vi "TPNT_UpdateDevice.vi"(5 "UTC":bool, 6 "mailserver":string="localhost", 7 "tpnt_logfile":path, 8 "error in (no error)":errorcluster, 10 "Device In":T1={"device"="", "devupdate"=0.0, "next_update"=0, "devinterface"="", "TPs"=[], "Alarms"=TRUE, "monitor"=TRUE, "log sep"=""} {"TPs"."Log"."updaterate" format="%.2f"; "TPs"."Samples"."Values" format="%.2f"; "TPs"."Samples"."samples" min=1 step=1; "TPs"."Limits"."Nominal" format="%.2f"; "TPs"."Limits"."Upper" format="%.2f"; "TPs"."Limits"."Lower" format="%.2f"; "TPs"."update_rate" format="%.2f"; "devupdate" format="%.2f"}) -> (0 "error out":errorcluster, 2 "Device IOut":T1={"device"="", "devupdate"=0.0, "next_update"=0, "devinterface"="", "TPs"=[], "Alarms"=TRUE, "monitor"=TRUE, "log sep"=""} {"TPs"."Log"."updaterate" format="%.2f"; "TPs"."Samples"."Values" format="%.2f"; "TPs"."Samples"."samples" min=1 step=1; "TPs"."Limits"."Nominal" format="%.2f"; "TPs"."Limits"."Upper" format="%.2f"; "TPs"."Limits"."Lower" format="%.2f"; "TPs"."update_rate" format="%.2f"; "devupdate" format="%.2f"})   [LabVIEW 2016]
uses:
  TPNT_DeviceTPs.ctl
  TPNT_TP.ctl
  TPNT_Limits.ctl
  TPNT_Samples.ctl
  TPNT_Log.ctl
panel:
  in  "attempts":i32=2
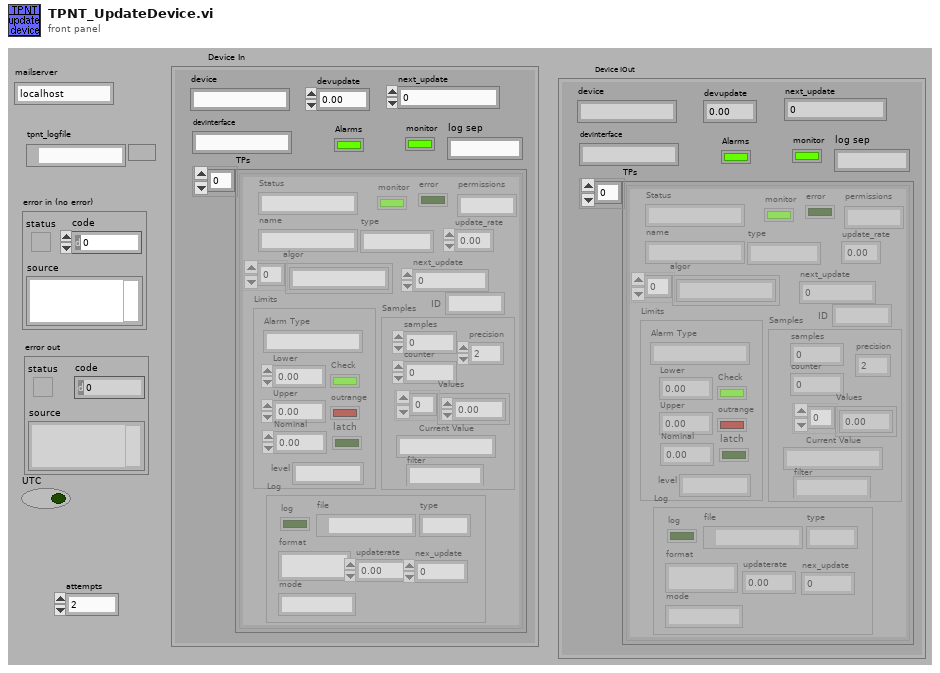
[diagram p1: front panel]
types:
  T1 = typedef "TPNT_DeviceTPs.ctl" = cluster{"device":string, "devupdate":dbl, "next_update":u32, "devinterface":string, "TPs":T2[], "Alarms":bool, "monitor":bool, "log sep":string}
  T2 = typedef "TPNT_TP.ctl" = cluster{"name":string, "type":string, "algor":string[], "update_rate":sgl, "Limits":T3, "Samples":T4, "next_update":u32, "Status":string, "monitor":bool, "error":bool, "Log":T5, "permissions":string, "ID":string}
  T3 = typedef "TPNT_Limits.ctl" = cluster{"Alarm Type":string, "Lower ":dbl, "Upper":dbl, "Nominal":dbl, "outrange":bool, "Check":bool, "latch":bool, "level":string}
  T4 = typedef "TPNT_Samples.ctl" = cluster{"samples":i32, "counter":i32, "Values":dbl[], "Current Value":string, "filter":string, "precision":u8}
  T5 = typedef "TPNT_Log.ctl" = cluster{"log":bool, "file":path, "type":string, "format":string, "updaterate":dbl, "nex_update":u32, "mode":string}
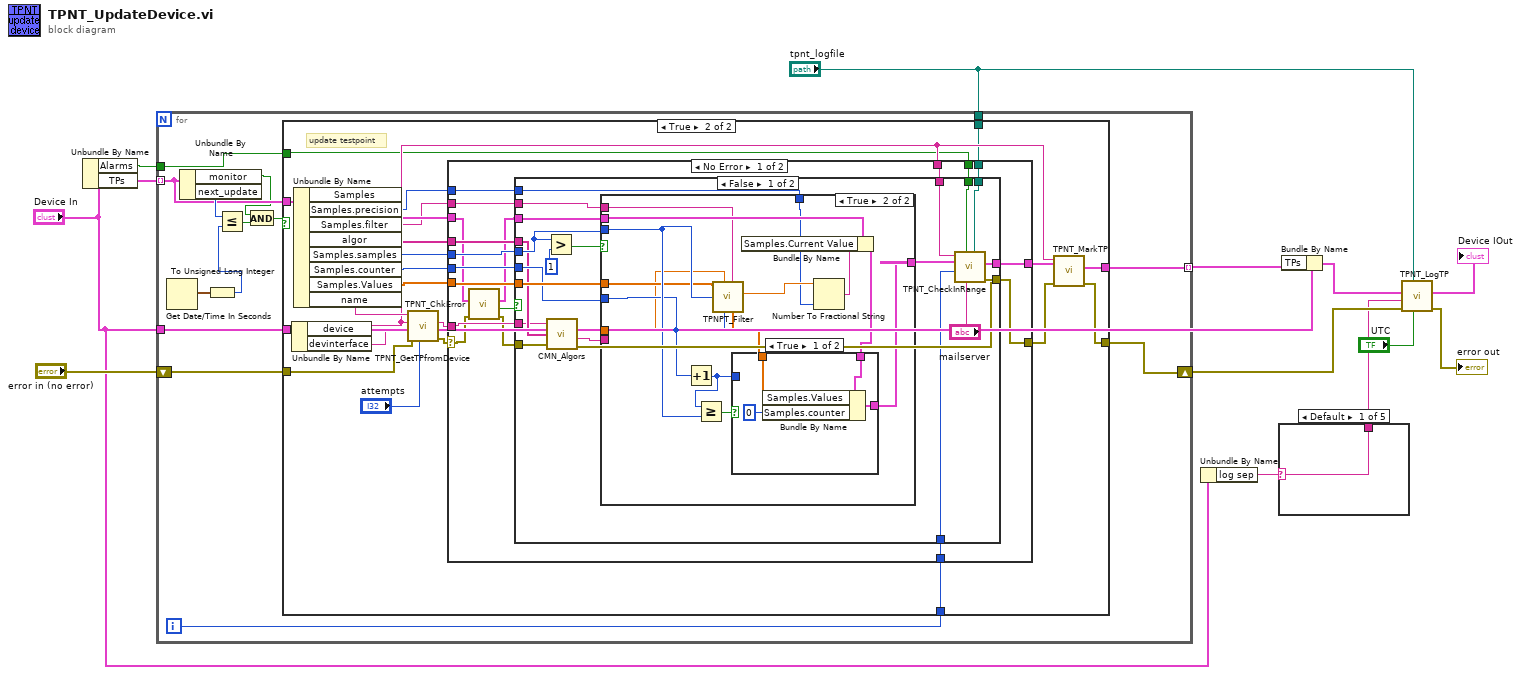
[diagram p0: block diagram]
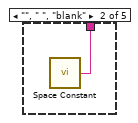
[diagram p2: hidden frame]
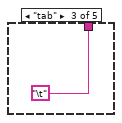
[diagram p3: hidden frame]
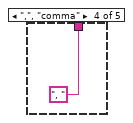
[diagram p4: hidden frame]
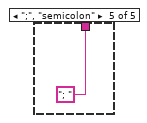
[diagram p5: hidden frame]
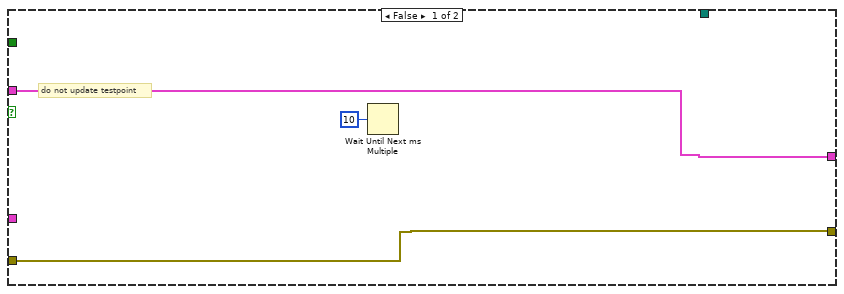
[diagram p6: hidden frame]
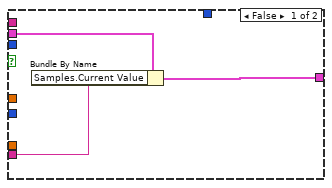
[diagram p7: hidden frame]
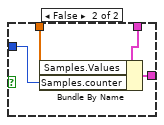
[diagram p8: hidden frame]
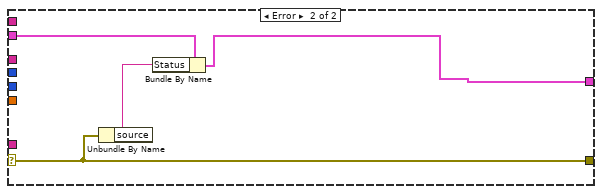
[diagram p10: hidden frame]
diagram:
  n1 = Unbundle By Name("Device In") -> ("Alarms"=w6:bool, "TPs"=w13:T2[])
  n2 = for {
    tunnel: w13 -> [w26] mode=indexing
    tunnel: "Device In" -> [w23]
    shift-right: [w24] -> w9
    shift-left: "error in (no error)" -> [w25]
    tunnel: [w22] -> w11 mode=indexing
    tunnel: w6 -> [w21]
    tunnel: "tpnt_logfile" -> [w15]
    i -> [w14]
    n3 = Get Date/Time In Seconds() -> (seconds since 1Jan1904=w17:timestamp)
    n4 = Unbundle By Name(w26) -> ("monitor"=w18:bool, "next_update"=w27:u32)
    n5 = To Unsigned Long Integer(number=w17) -> (unsigned 32bit integer=w16:u32)
    n6 = Less Or Equal?(x=w27, y=w16) -> (x <= y?=w20:bool)
    n7 = And(x=w18, y=w20) -> (x .and. y?=w19:bool)
    n8 = case shown="True" w19 {
      tunnel: w26 -> [w28 w35]
      tunnel: w23 -> [_ w52]
      tunnel: w25 -> [w29 w50]
      tunnel: [w29 w40] -> w24
      tunnel: [w28 w39] -> w22
      tunnel: w21 -> [_ w37]
      tunnel: w15 -> [_ w32]
      tunnel: w14 -> [_ w31]
      frame False {
        # "do not update testpoint"
        n9 = Wait Until Next ms Multiple(millisecond multiple=u32 10) -> ()  [unwired: 1 out]
      }
      frame True {
        # "update testpoint"
        n10 = Unbundle By Name(w52) -> ("device"=w38:string, "devinterface"=w51:string)
        n11 = Unbundle By Name(w35) -> ("Samples.precision"=w33:u8, "Samples.filter"=w34:string, "algor"=w36:string[], "Samples.samples"=w44:i32, "Samples.counter"=w45:i32, "Samples.Values"=w46:dbl[], "name"=w48:string)  [unwired: 1 out]
        n12 = call "TPNT_GetTPfromDevice.vi"("attempts"="attempts", "error in (no error)"=w50, "device interface"=w51, "device name"=w38, "testpoint name"=w48) -> ("error out"=w47:errorcluster, "value out"=w43:string)  [unwired: 5 out]
        n13 = case shown="No Error" w47 {
          selector: w47 -> [w61 w123]
          tunnel: [w67 w123] -> w41
          tunnel: w46 -> [w70 _]
          tunnel: w45 -> [w69 _]
          tunnel: w44 -> [w68 _]
          tunnel: w43 -> [w62 _]
          tunnel: w35 -> [w59 w121]
          tunnel: [w66 w120] -> w42
          tunnel: w38 -> [w65 _]
          tunnel: w37 -> [w64 _]
          tunnel: w36 -> [w63 _]
          tunnel: w34 -> [w56 _]
          tunnel: w33 -> [w55 _]
          tunnel: w32 -> [w54 _]
          tunnel: w31 -> [w53 _]
          frame No Error {
            n14 = call "TPNT_ChkError.vi"("error in (no error)"=w61, "testpoint In"=w59) -> ("error out"=w60:errorcluster, "error"=w57:bool, "testpoint out"=w58:T2)  [unwired: 7 out]
            n15 = case shown="False" w57 {
              tunnel: w70 -> [w92 _]
              tunnel: w69 -> [w91 _]
              tunnel: w58 -> [w88 w119]
              tunnel: w68 -> [w87 _]
              tunnel: [w85 w118] -> w67
              tunnel: [w84 w119] -> w66
              tunnel: w65 -> [w83 _]
              tunnel: w64 -> [w82 _]
              tunnel: w60 -> [w81 w118]
              tunnel: w63 -> [w79 _]
              tunnel: w62 -> [w76 _]
              tunnel: w56 -> [w75 _]
              tunnel: w55 -> [w74 _]
              tunnel: w54 -> [w72 _]
              tunnel: w53 -> [w71 _]
              frame False {
                n16 = Greater?(x=w87, y=1) -> (0:w89:bool)
                n17 = call "CMN_Algors.vi"("ValueIn"=w76, "algors"=w79, "error in (no error)"=w81) -> ("Value out"=w77:sgl, "string value"=w78:string, "error out"=w80:errorcluster)  [unwired: 2 in, 3 out]
                n18 = case shown="True" w89 {
                  tunnel: w92 -> [_ w101]
                  tunnel: w91 -> [_ w102]
                  tunnel: w88 -> [w95 w98]
                  tunnel: w87 -> [_ w107]
                  tunnel: w78 -> [w94 _]
                  tunnel: [w93 w104] -> w86
                  tunnel: w77 -> [_ w99]
                  tunnel: w75 -> [_ w97]
                  tunnel: w74 -> [_ w96]
                  frame False {
                    n19 = Bundle By Name(cluster=w95, "Samples.Current Value"=w94) -> (w93:T2)
                  }
                  frame True {
                    n20 = Increment(x=w102) -> (x+1=w103:i32)
                    n21 = Greater Or Equal?(x=w103, y=w107) -> (x >= y?=w106:bool)
                    n22 = call "TPNPT_Filter.vi"("Values"=w101, "last value"=w99, "Number of samples"=w107, "index"=w102, "filter"=w97) -> ("output"=w109:dbl, "Values out"=w100:dbl[])  [unwired: 1 in, 3 out]
                    n23 = Number To Fractional String(number=w109, precision (6)=w96) -> (F-format string=w108:string)  [unwired: 2 out]
                    n24 = Bundle By Name(cluster=w98, "Samples.Current Value"=w108) -> (w105:T2)
                    n25 = case shown="True" w106 {
                      tunnel: w100 -> [w113 w117]
                      tunnel: w105 -> [w112 w116]
                      tunnel: [w111 w115] -> w104
                      tunnel: w103 -> [_ w114]
                      frame True {
                        n26 = Bundle By Name(cluster=w112, "Samples.Values"=w113, "Samples.counter"=0) -> (w111:T2)
                      }
                      frame False {
                        n27 = Bundle By Name(cluster=w116, "Samples.Values"=w117, "Samples.counter"=w114) -> (w115:T2)
                      }
                    }
                  }
                }
                n28 = call "TPNT_CheckInRange.vi"("tpnt_logfile"=w72, "mailserver"="mailserver", "check alarms"=w82, "error in (no error)"=w80, "index in"=w71, "testpoint In"=w86, "device"=w83) -> ("error out"=w85:errorcluster, "testpoint Out"=w84:T2)  [unwired: 3 out]
              }
              frame True {
              }
            }
          }
          frame Error {
            n29 = Unbundle By Name(w123) -> ("source"=w122:string)
            n30 = Bundle By Name(cluster=w121, "Status"=w122) -> (w120:T2)
          }
        }
        n31 = call "TPNT_MarkTP.vi"("error in (no error)"=w41, "testpoint In"=w42, "device"=w38) -> ("error out"=w40:errorcluster, "testpoint Out"=w39:T2)  [unwired: 7 out]
      }
    }
  }
  n32 = Unbundle By Name("Device In") -> ("log sep"=w4:string)
  n33 = case shown="Default" w4 {
    selector: w4 -> [w124 _ _ _ _]
    tunnel: [w124 w125 "\t" ", " ("String") "; " ("String")] -> w3
    frame Default {
    }
    frame "", " ", "blank" {
      n34 = call <vilib>:"Space Constant.vi"() -> ("String"=w125:string)
    }
    frame "tab" {
    }
    frame ",", "comma" {
    }
    frame ";", "semicolon" {
    }
  }
  n35 = Bundle By Name(cluster="Device In", "TPs"=w11) -> (w10:T1)
  n36 = call "TPNT_LogTP.vi"("UTC"="UTC", "tpnt_logfile"="tpnt_logfile", "error in (no error)"=w9, "tp separator"=w3, "Device"=w10) -> ("error out"=→"error out":errorcluster, "Devices out"=→"Device IOut":T1)  [unwired: 5 out]
